vi "Sub_Set_fixed_Current_Measurement.vi"(2 "error in":errorcluster, 3 "i":i32, 4 "AgB29xxLib.IAgB29xx2":refnum<k7>) -> (0 "error out":errorcluster, 1 "AgB29xxLib.IAgB29xx2 2":refnum<k7>)   [LabVIEW 2009]
panel:
  # "Sub VI: Set Trigger Condition"
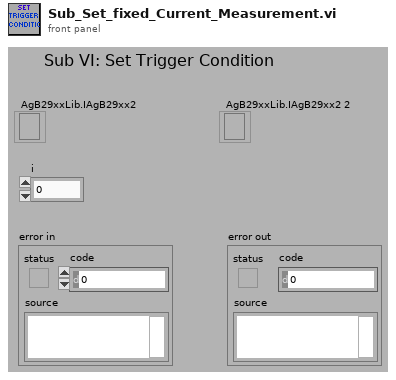
[diagram p1: front panel]
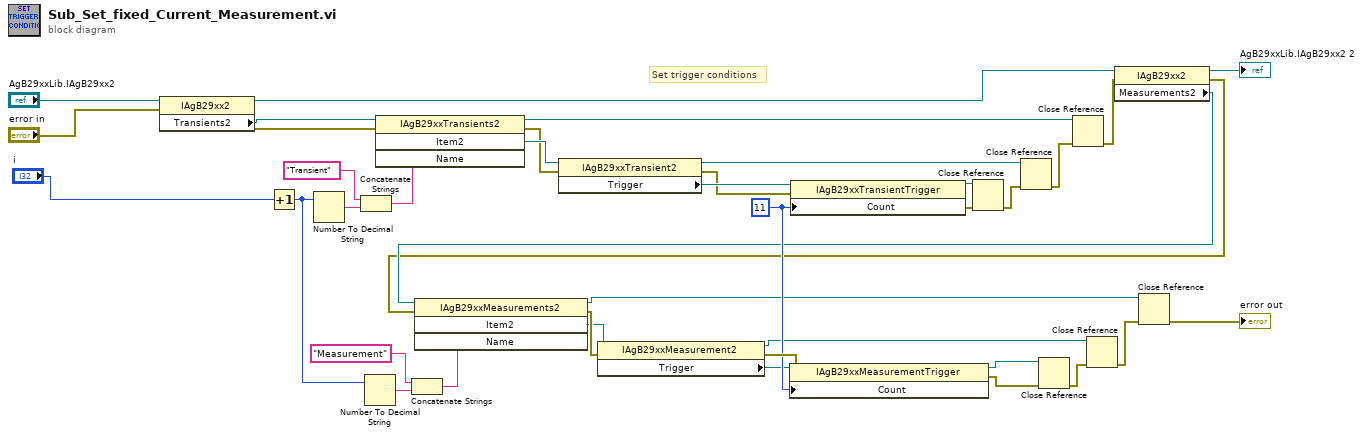
[diagram p0: block diagram]
diagram:
  w13 = u32 11 ("milliseconds to wait")
  # "Set trigger conditions"
  n1 = property class="IAgB29xx2"(reference="AgB29xxLib.IAgB29xx2", error in="error in") -> (reference out=w34:refnum<k7>, error out=w36:errorcluster, "Transients2"=w35:refnum<k7>)
  n2 = Increment(x="i") -> (x+1=w15:i32)
  n3 = Number To Decimal String(number=w15) -> (decimal integer string=w30:string)  [unwired: 1 in]
  n4 = Concatenate Strings("Transient" ("string"), w30) -> (w28:string)
  n5 = Number To Decimal String(number=w15) -> (decimal integer string=w19:string)  [unwired: 1 in]
  n6 = invoke class="IAgB29xxTransients2" method="Item2"(reference=w35, error in=w36, "Name"=w28) -> (reference out=w20:refnum<k7>, error out=w25:errorcluster, "Item2"=w31:refnum<k7>)  [unwired: 1 in, 1 out]
  n7 = Concatenate Strings("Measurement" ("string"), w19) -> (w17:string)
  n8 = property class="IAgB29xxTransient2"(reference=w31, error in=w25) -> (reference out=w22:refnum<k7>, error out=w26:errorcluster, "Trigger"=w27:refnum<k7>)
  n9 = property class="IAgB29xxTransientTrigger"(reference=w27, error in=w26, "Count"=w13) -> (reference out=w24:refnum<k7>, error out=w12:errorcluster)
  n10 = Close Reference(reference=w24, error in (no error)=w12) -> (error out=w23:errorcluster)
  n11 = Close Reference(reference=w22, error in (no error)=w23) -> (error out=w21:errorcluster)
  n12 = Close Reference(reference=w20, error in (no error)=w21) -> (error out=w11:errorcluster)
  n13 = property class="IAgB29xx2"(reference=w34, error in=w11) -> (reference out=→"AgB29xxLib.IAgB29xx2 2":refnum<k7>, error out=w9:errorcluster, "Measurements2"=w10:refnum<k7>)
  n14 = invoke class="IAgB29xxMeasurements2" method="Item2"(reference=w10, error in=w9, "Name"=w17) -> (reference out=w3:refnum<k7>, error out=w16:errorcluster, "Item2"=w1:refnum<k7>)  [unwired: 1 in, 1 out]
  n15 = property class="IAgB29xxMeasurement2"(reference=w1, error in=w16) -> (reference out=w4:refnum<k7>, error out=w14:errorcluster, "Trigger"=w2:refnum<k7>)
  n16 = property class="IAgB29xxMeasurementTrigger"(reference=w2, error in=w14, "Count"=w13) -> (reference out=w5:refnum<k7>, error out=w6:errorcluster)
  n17 = Close Reference(reference=w5, error in (no error)=w6) -> (error out=w7:errorcluster)
  n18 = Close Reference(reference=w4, error in (no error)=w7) -> (error out=w8:errorcluster)
  n19 = Close Reference(reference=w3, error in (no error)=w8) -> (error out=→"error out":errorcluster)
